vi "6762_Auto.vi"() -> ()   [LabVIEW 2017]
doc: "This VI is called when autonomous begins, and will automatically be terminated when autonomous ends. You can carry out timed or sensor driven robot movement independently without needing to return to the caller."
uses:
  <vilib>/Rock Robotics/Network Tables/NT Write Numeric Array.vi
  Robot Global Data.vi
  <vilib>/Rock Robotics/Network Tables/NT Read String.vi
panel:
  out "Current Movement, for debugging":T1 {"Y Joystick Value" scale=1.0..-1.0; "X Joystick Value" scale=-1.0..1.0}
  in  "Array of robot movements":T2(array[cluster])=[{"X Joystick Value"=0.39393939393939403, "Y Joystick Value"=0.0, "Delay (sec)"=1.0, "Movement Name"="turn"}, {"X Joystick Value"=-0.3737373737373737, "Y Joystick Value"=0.0, "Delay (sec)"=1.0, "Movement Name"="turn back"}] {"Y Joystick Value" scale=1.0..-1.0; "X Joystick Value" scale=-1.0..1.0}
  # "Be sure to right-click and choose Data Operations>>Make Current Value default if you want to save the array values with the VI"
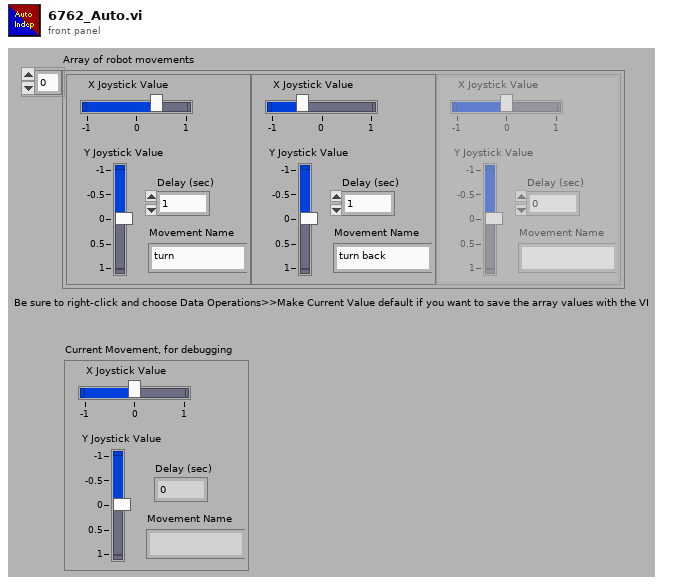
[diagram p1: front panel]
types:
  T1 = cluster{"X Joystick Value":dbl, "Y Joystick Value":dbl, "Delay (sec)":dbl, "Movement Name":string}
  T2 = cluster{"X Joystick Value":dbl, "Y Joystick Value":dbl, "Delay (sec)":dbl, "Movement Name":string}[]
  T3 = typedef "WPI_JoystickDevRef.ctl" = cluster{"Device":T4}
  T4 = typedef "WPI_JoystickDeviceEnum.ctl" = enum16{"USB 0", "USB 1", "USB 2", "USB 3", "USB 4", "USB 5"}
  T5 = enum16{"Forward", "VisionTrack00", "VisionTrackingAtEdge", "ResetTime", "TimedForward", "Stop"}
  T6 = enum16{"Start", "Vision Tracking Center", "ResetTime", "Time Forward", "drop block", "Time Reset", "Back up", "Time reset", "go Left or Right", "time Reset", "go straight", "Stop"}
  T7 = typedef "WPI_RobotDriveDevRef.ctl" = cluster{"DevStatus":errorcluster, "Motors[]":T8[], "Square Inputs":bool, "Max Output":dbl}
  T8 = typedef "WPI_MotorControlDeviceRef.ctl" = cluster{"DeviceStatus":errorcluster, "Type":T9, "PWM":cluster{"PWM Channel":T10, "DeadBand":T11}, "CAN":cluster{"Device Number":u8, "SetOutput VI Ref":variant, "GetOutput VI Ref":variant, "Enable VI Ref":variant, "Disable VI Ref":variant, "Data":variant}, "Invert":bool, "DIO PWM":cluster{"PWM \"Enable\" Channel":T10, "DIOChannel":T12, "PWM Rate":dbl}}
  T9 = typedef "WPI_MotorControlType.ctl" = enum16{"PWM", "CAN", "DIO PWM"}
  T10 = typedef "FPGA_DIOPWMChannel.ctl" = enum8{"PWM 0", "PWM 1", "PWM 2", "PWM 3", "PWM 4", "PWM 5", "PWM 6", "PWM 7", "PWM 8", "PWM 9", "PWM MXP 0", "PWM MXP 1", "PWM MXP 2", "PWM MXP 3", "PWM MXP 4", "PWM MXP 5", "PWM MXP 6", "PWM MXP 7", "PWM MXP 8", "PWM MXP 9", "Invalid"}
  T11 = typedef "WPI_PWMDeadband.ctl" = cluster{"Name":string, "maxPositivePwm":i32, "minPositivePwm":i32, "centerPwm":i32, "maxNegativePwm":i32, "minNegativePwm":i32, "angularRange":u16}
  T12 = typedef "FPGA_DIOChannel.ctl" = enum8{"DIO 0", "DIO 1", "DIO 2", "DIO 3", "DIO 4", "DIO 5", "DIO 6", "DIO 7", "DIO 8", "DIO 9", "DIO MXP 0", "DIO MXP 1", "DIO MXP 2", "DIO MXP 3", "DIO MXP 4", "DIO MXP 5", "DIO MXP 6", "DIO MXP 7", "DIO MXP 8", "DIO MXP 9", "DIO MXP 10", "DIO MXP 11", "DIO MXP 12", "DIO MXP 13", "DIO MXP 14", "DIO MXP 15", "SPI Port CS1", "SPI Port CS2", "SPI Port CS3", "SPI Port MISO", "SPI Port MOSI", "Invalid"}
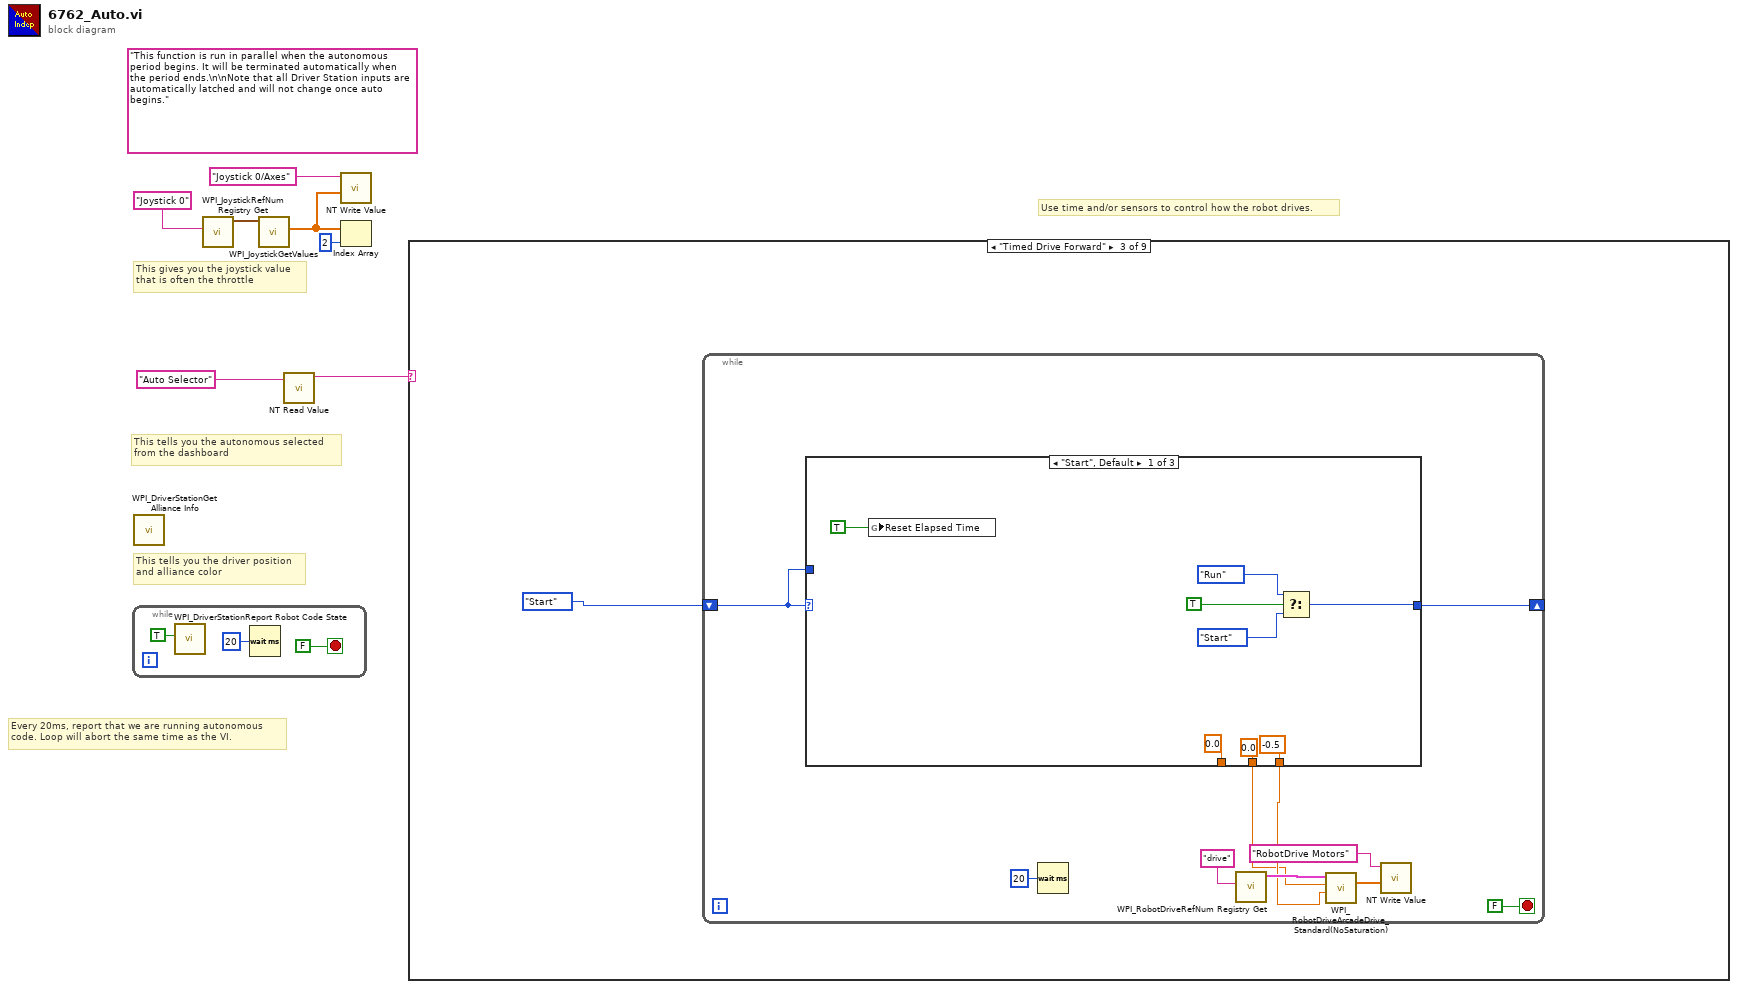
[diagram p0: block diagram]
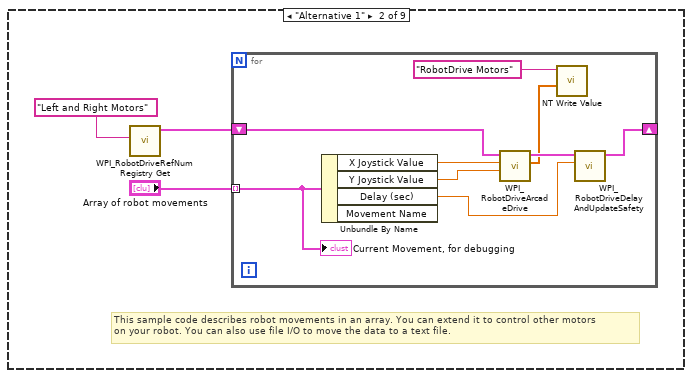
[diagram p3: hidden frame]
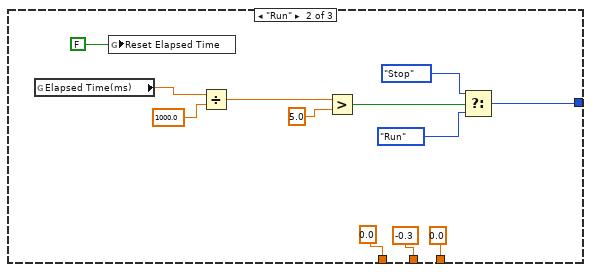
[diagram p4: hidden frame]
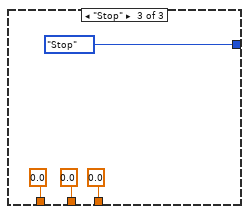
[diagram p5: hidden frame]
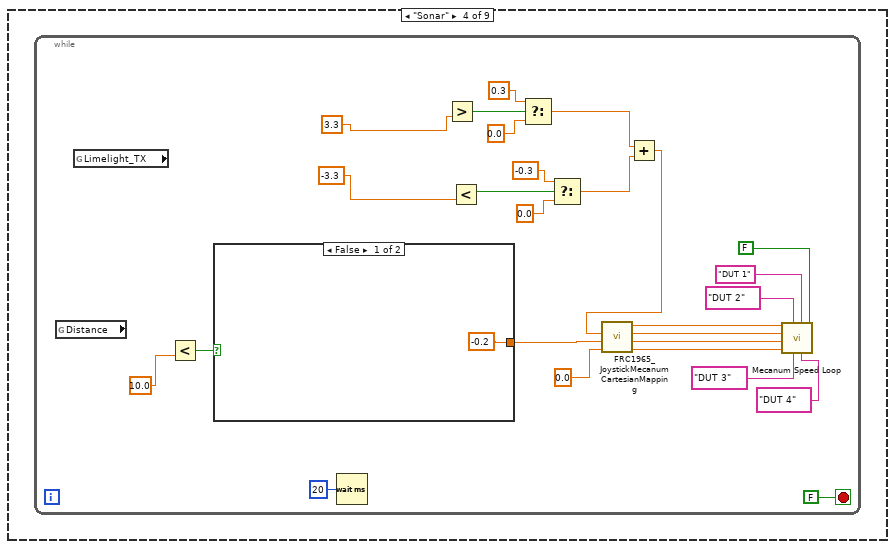
[diagram p6: hidden frame]
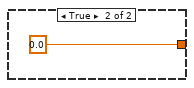
[diagram p7: hidden frame]
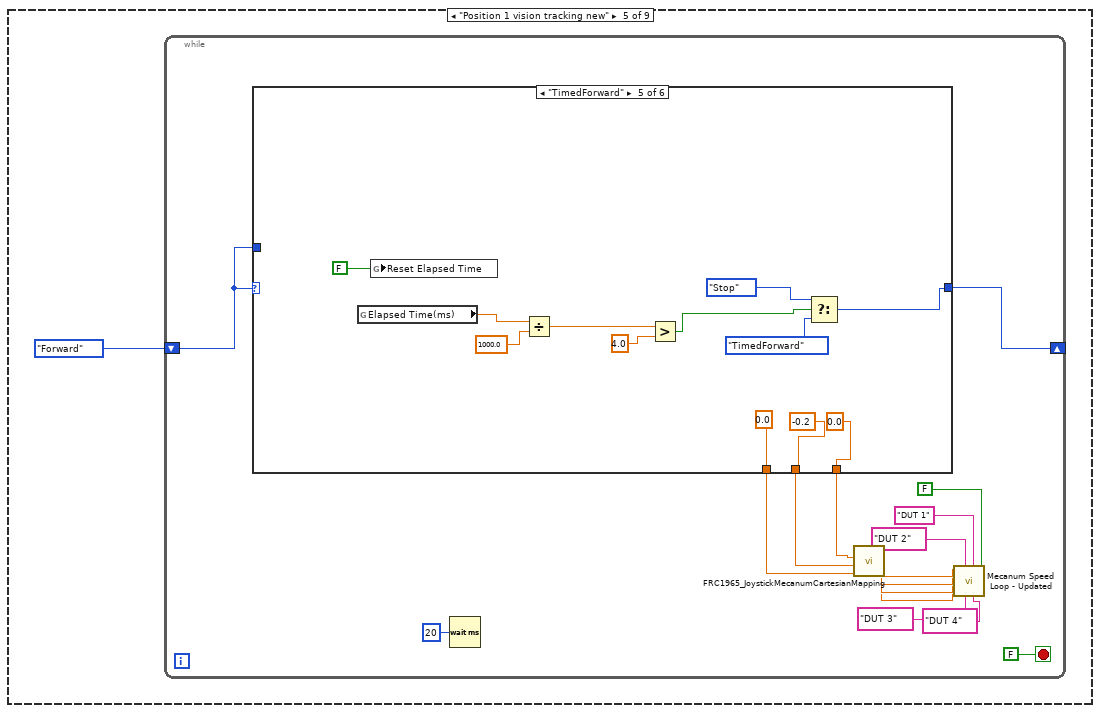
[diagram p8: hidden frame]
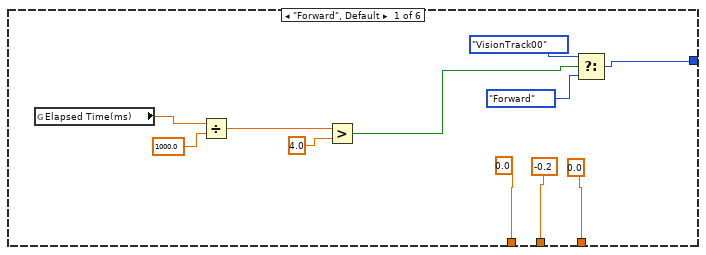
[diagram p9: hidden frame]
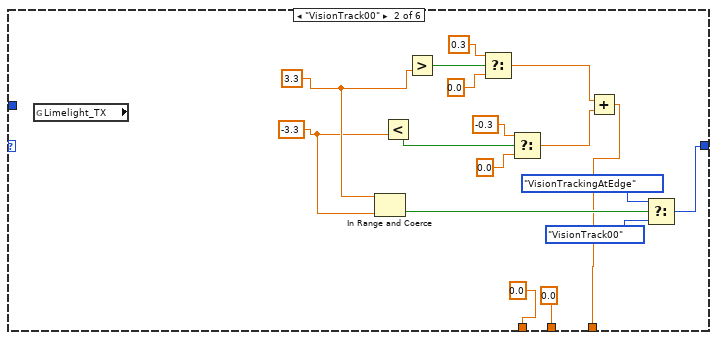
[diagram p10: hidden frame]
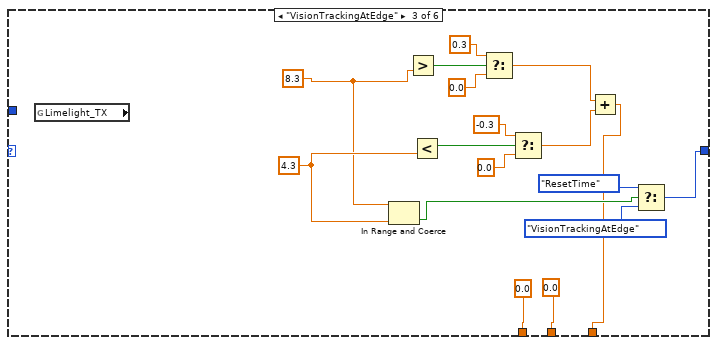
[diagram p11: hidden frame]
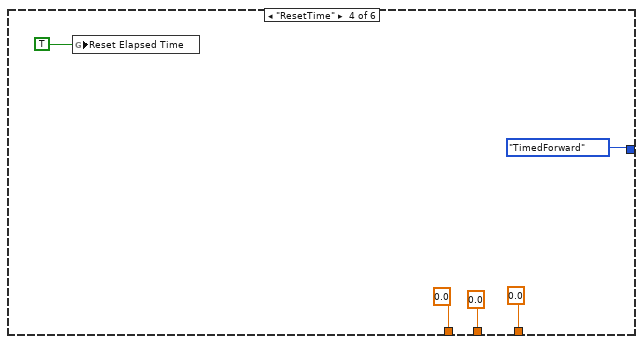
[diagram p12: hidden frame]
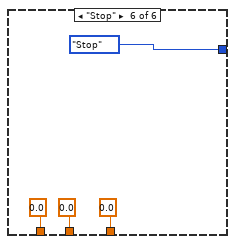
[diagram p13: hidden frame]
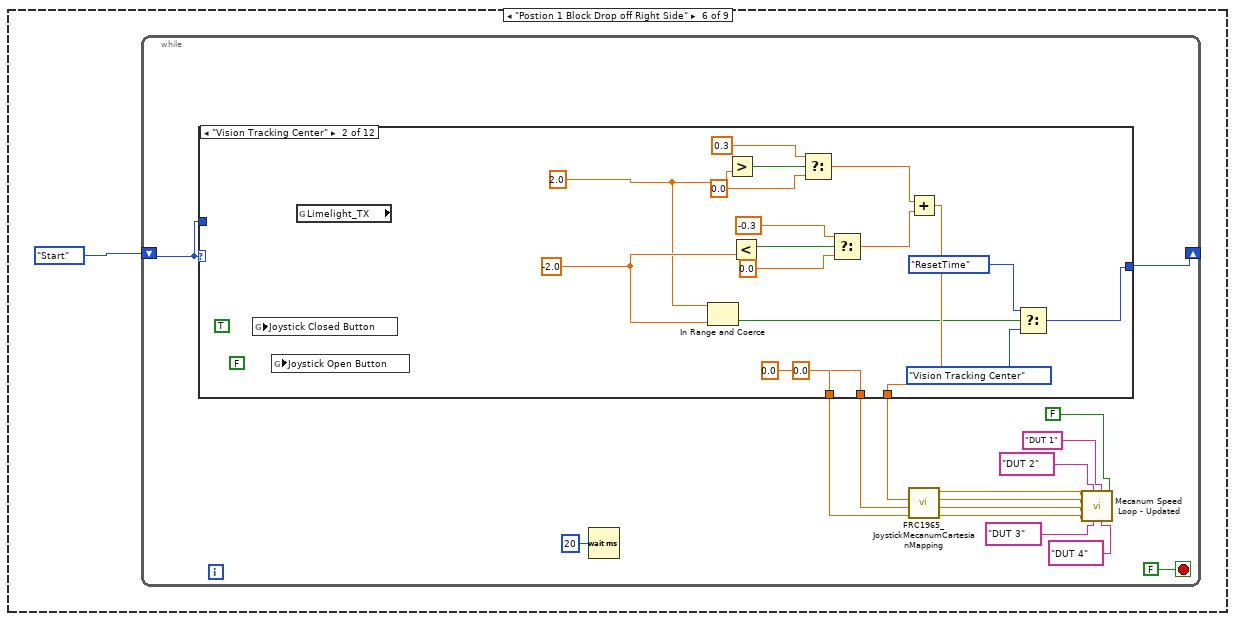
[diagram p14: hidden frame]
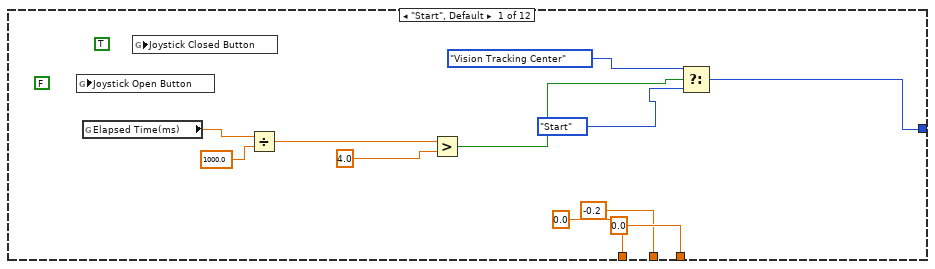
[diagram p15: hidden frame]
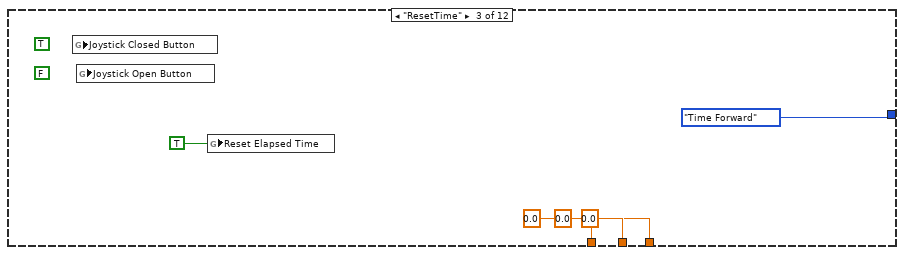
[diagram p16: hidden frame]
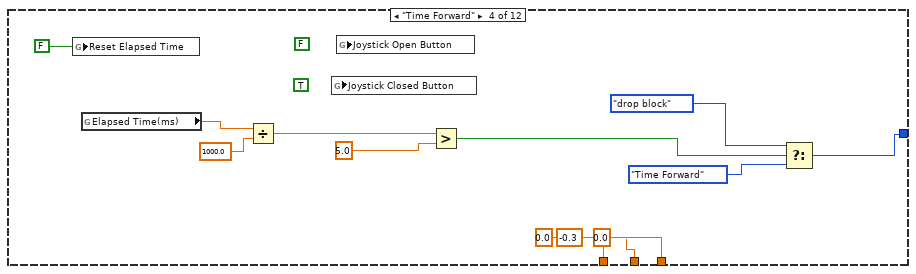
[diagram p17: hidden frame]
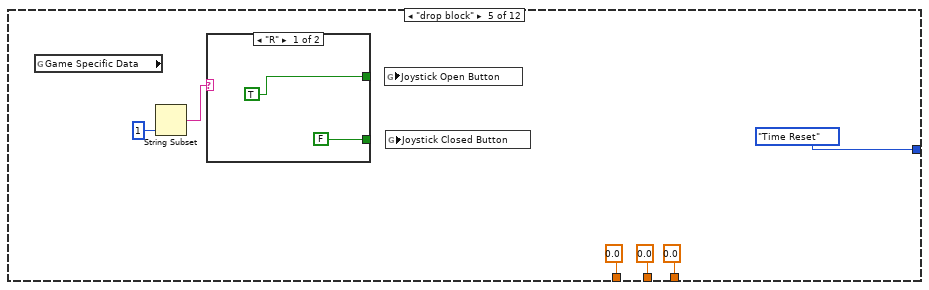
[diagram p18: hidden frame]
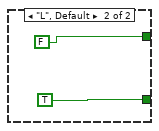
[diagram p19: hidden frame]
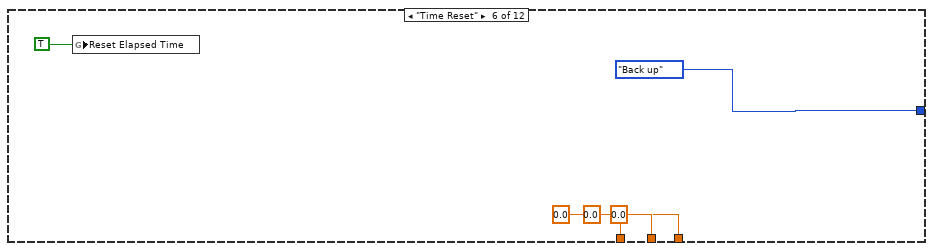
[diagram p20: hidden frame]
diagram:
  (unwired) "This function is run in parallel when the autonomous period begins. It will be terminated automatically when the period ends.\n\nNote that all Driver Station inputs are automatically latched and will not change once auto begins."
  # "Use time and/or sensors to control how the robot drives."
  # "This tells you the autonomous selected\nfrom the dashboard"
  # "Every 20ms, report that we are running autonomous\ncode. Loop will abort the same time as the VI."
  # "This gives you the joystick value\nthat is often the throttle"
  # "This tells you the driver position\nand alliance color"
  n1 = while {
    stop <- FALSE stop-if-true
    n2 = call <vilib>:"WPI_DriverStationReport Robot Code State.vi"("Autonomous"=TRUE) -> ()  [unwired: 10 in, 1 out]
    n3 = Wait (ms)(milliseconds to wait=u32 20) -> ()  [unwired: 1 out]
  }
  n4 = call <vilib>:"WPI_DriverStationGet Alliance Info.vi"() -> ()  [unwired: 12 out]
  n5 = call <vilib>:"WPI_JoystickRefNum Registry Get.vi"("refnum name"="Joystick 0") -> ("JoystickDevRef"=w6:T3)  [unwired: 1 in, 9 out]
  n6 = call <vilib>:"WPI_JoystickGetValues.vi"("JoystickDevRef"=w6) -> ("Axes"=w2:dbl[])  [unwired: 6 in, 4 out]
  n7 = call-poly <vilib>:"NT Read Value.vi"("Name"="Auto Selector") -> ("String"=w3:string)  [unwired: 9 in, 1 out]
  n8 = call-poly <vilib>:"NT Write Value.vi"("Numeric Array"=w2, "Name"="Joystick 0/Axes") -> ()  [unwired: 9 in, 1 out]
  n9 = Index Array(array=w2, index=2) -> ()  [unwired: 1 out]
  n10 = case shown="\"Timed Drive Forward\"" w3 {
    frame Default {
      # "You can put your main auto here, or you can right-click on the case and make any\nother frame be the default case."
      # "This is the frame that will execute if no selection is made, or if it is not recognized"
    }
    frame "Alternative 1" {
      # "This sample code describes robot movements in an array. You can extend it to control other motors\non your robot. You can also use file I/O to move the data to a text file."
      n11 = call <vilib>:"WPI_RobotDriveRefNum Registry Get.vi"("refnum name"="Left and Right Motors") -> ("RobotDriveDevRef"=w12:T7)  [unwired: 1 in, 9 out]
      n12 = for {
        shift-right: [w20] -> _
        shift-left: w12 -> [w21]
        tunnel: "Array of robot movements" -> [w16] mode=indexing
        n13 = Unbundle By Name(w16) -> ("X Joystick Value"=w19:dbl, "Y Joystick Value"=w18:dbl, "Delay (sec)"=w17:dbl)  [unwired: 1 out]
        n14 = call-poly <vilib>:"WPI_RobotDriveArcadeDrive.vi"("Y axis value"=w18, "X axis value"=w19, "RobotDriveDevRef"=w21) -> ("Motor Values"=w14:dbl[], "RobotDriveDevRef"=w22:T7)  [unwired: 1 in, 6 out]
        n15 = call-poly <vilib>:"NT Write Value.vi"("Numeric Array"=w14, "Name"="RobotDrive Motors") -> ()  [unwired: 9 in, 1 out]
        n16 = call <vilib>:"WPI_RobotDriveDelayAndUpdateSafety.vi"("Delay (s)"=w17, "RobotDriveDevRef"=w22) -> ("RobotDriveDevRef 2"=w20:T7)  [unwired: 8 in, 1 out]
        "Current Movement, for debugging" <- w16
      }
    }
    frame "Timed Drive Forward" {
      n17 = while {
        shift-right: [w33] -> _
        shift-left: enum16{"Start", "Run", "Stop"}."Start" ("Enum") -> [w32]
        stop <- FALSE stop-if-true
        n18 = case shown="\"Start\", Default" w32 {
          tunnel: [0.0 ("X") 0.0 ("X") 0.0 ("X")] -> _
          tunnel: [0.0 ("X") -0.3 ("X") 0.0 ("X")] -> w24
          tunnel: [-0.5 ("X") 0.0 ("X") 0.0 ("X")] -> w25
          tunnel: [w35 w48 enum16{"Start", "Run", "Stop"}."Stop" ("Enum")] -> w33
          tunnel: w32 -> [_ _ _]
          frame "Start", Default {
            n19 = global write "Robot Global Data.vi" "Reset Elapsed Time"(TRUE ("Reset Elapsed Time")) -> ()
            n20 = Select(t=enum16{"Start", "Run", "Stop"}."Run" ("Enum"), s=TRUE, f=enum16{"Start", "Run", "Stop"}."Start" ("Enum")) -> (s? t:f=w35:enum16{"Start", "Run", "Stop"})
          }
          frame "Run" {
            n21 = global read "Robot Global Data.vi" "Elapsed Time(ms)"() -> (w46:dbl)
            n22 = global write "Robot Global Data.vi" "Reset Elapsed Time"(FALSE ("Reset Elapsed Time")) -> ()
            n23 = Divide(x=w46, y=1000.0) -> (x/y=w47:dbl)
            n24 = Greater?(x=w47, y=5.0) -> (0:w43:bool)
            n25 = Select(t=enum16{"Start", "Run", "Stop"}."Stop" ("Enum"), s=w43, f=enum16{"Start", "Run", "Stop"}."Run" ("Enum")) -> (s? t:f=w48:enum16{"Start", "Run", "Stop"})
          }
          frame "Stop" {
          }
        }
        n26 = Wait (ms)(milliseconds to wait=u32 20) -> ()  [unwired: 1 out]
        n27 = call <vilib>:"WPI_RobotDriveRefNum Registry Get.vi"("refnum name"="drive") -> ("RobotDriveDevRef"=w28:T7)  [unwired: 1 in, 9 out]
        n28 = call <vilib>:"WPI_RobotDriveArcadeDrive_Standard(NoSaturation).vi"("Y axis value"=w25, "X axis value"=w24, "RobotDriveDevRef"=w28) -> ("Motor Values"=w27:dbl[])  [unwired: 1 in, 7 out]
        n29 = call-poly <vilib>:"NT Write Value.vi"("Numeric Array"=w27, "Name"="RobotDrive Motors") -> ()  [unwired: 9 in, 1 out]
      }
    }
    frame "Sonar" {
      n30 = while {
        stop <- FALSE stop-if-true
        n31 = global read "Robot Global Data.vi" "Distance"() -> ()  [unwired: 1 out]
        n32 = global read "Robot Global Data.vi" "Limelight_TX"() -> ()  [unwired: 1 out]
        n33 = Less?(y=10.0) -> (x < y?=w82:bool)  [unwired: 1 in]
        n34 = case shown="False" w82 {
          tunnel: [-0.2 ("y") 0.0 ("y")] -> w72
          frame False {
          }
          frame True {
          }
        }
        n35 = Wait (ms)(milliseconds to wait=u32 20) -> ()  [unwired: 1 out]
        n36 = Greater?(y=3.3 ("upper limit")) -> (0:w67:bool)  [unwired: 1 in]
        n37 = Less?(y=-3.3 ("lower limit")) -> (x < y?=w62:bool)  [unwired: 1 in]
        n38 = Select(t=0.3, s=w67, f=0.0) -> (s? t:f=w61:dbl)
        n39 = Select(t=-0.3, s=w62, f=0.0) -> (s? t:f=w60:dbl)
        n40 = Add(x=w61, y=w60) -> (x+y=w59:dbl)
        n41 = call "FRC1965_JoystickMecanumCartesianMapping.vi"("Rotation"=0.0, "Y"=w72, "X"=w59) -> ("Rear Right"=w73:dbl, "Rear Left"=w74:dbl, "Front Right"=w75:dbl, "Front Left"=w76:dbl)  [unwired: 5 in]
        n42 = call "Mecanum Speed Loop.vi"("Closed Loop Select"=FALSE, "DUT Number 4"="DUT 4" ("refnum name"), "DUT Number 1"="DUT 1" ("refnum name"), "DUT Number 3"="DUT 3" ("refnum name"), "DUT Number 2"="DUT 2" ("refnum name"), "Rear Right"=w73, "Rear Left"=w74, "Front Right"=w75, "Front Left"=w76) -> ()  [unwired: 3 in]
      }
    }
    frame "Position 1 vision tracking new" {
      n43 = while {
        shift-right: [w90] -> _
        shift-left: T5."Forward" ("State") -> [w89]
        stop <- FALSE stop-if-true
        n44 = case shown="\"TimedForward\"" w89 {
          tunnel: [-0.2 ("Y") 0.0 ("Rotation") 0.0 ("Rotation") 0.0 ("Rotation") -0.2 ("Rotation") 0.0 ("Rotation")] -> w93
          tunnel: [0.0 ("Rotation") 0.0 ("Rotation") 0.0 ("Rotation") 0.0 ("Rotation") 0.0 ("Rotation") 0.0 ("Rotation")] -> w92
          tunnel: [0.0 ("X") w117 w134 0.0 ("Rotation") 0.0 ("Rotation") 0.0 ("Rotation")] -> w91
          tunnel: [w103 w114 w131 T5."TimedForward" ("State") w153 T5."Stop" ("State")] -> w90
          tunnel: w89 -> [_ _ _ _ _ _]
          frame "Forward", Default {
            n45 = global read "Robot Global Data.vi" "Elapsed Time(ms)"() -> (w112:dbl)
            n46 = Divide(x=w112, y=1000.0) -> (x/y=w113:dbl)
            n47 = Greater?(x=w113, y=4.0) -> (0:w109:bool)
            n48 = Select(t=T5."VisionTrack00" ("State"), s=w109, f=T5."Forward" ("State")) -> (s? t:f=w103:T5)
          }
          frame "VisionTrack00" {
            w120 = -3.3 ("lower limit")
            w122 = 3.3 ("upper limit")
            n49 = global read "Robot Global Data.vi" "Limelight_TX"() -> ()  [unwired: 1 out]
            n50 = In Range and Coerce(upper limit=w122, lower limit=w120) -> (In Range?=w121:bool)  [unwired: 1 in, 1 out]
            n51 = Less?(y=w120) -> (x < y?=w125:bool)  [unwired: 1 in]
            n52 = Greater?(y=w122) -> (0:w130:bool)  [unwired: 1 in]
            n53 = Select(t=0.3, s=w130, f=0.0) -> (s? t:f=w124:dbl)
            n54 = Select(t=-0.3, s=w125, f=0.0) -> (s? t:f=w123:dbl)
            n55 = Add(x=w124, y=w123) -> (x+y=w117:dbl)
            n56 = Select(t=T5."VisionTrackingAtEdge" ("State"), s=w121, f=T5."VisionTrack00" ("State")) -> (s? t:f=w114:T5)
          }
          frame "VisionTrackingAtEdge" {
            w138 = 4.3 ("lower limit")
            w137 = 8.3 ("upper limit")
            n57 = global read "Robot Global Data.vi" "Limelight_TX"() -> ()  [unwired: 1 out]
            n58 = In Range and Coerce(upper limit=w137, lower limit=w138) -> (In Range?=w139:bool)  [unwired: 1 in, 1 out]
            n59 = Greater?(y=w137) -> (0:w147:bool)  [unwired: 1 in]
            n60 = Less?(y=w138) -> (x < y?=w142:bool)  [unwired: 1 in]
            n61 = Select(t=0.3, s=w147, f=0.0) -> (s? t:f=w141:dbl)
            n62 = Select(t=-0.3, s=w142, f=0.0) -> (s? t:f=w140:dbl)
            n63 = Add(x=w141, y=w140) -> (x+y=w134:dbl)
            n64 = Select(t=T5."ResetTime" ("State"), s=w139, f=T5."VisionTrackingAtEdge" ("State")) -> (s? t:f=w131:T5)
          }
          frame "ResetTime" {
            n65 = global write "Robot Global Data.vi" "Reset Elapsed Time"(TRUE ("Reset Elapsed Time")) -> ()
          }
          frame "TimedForward" {
            n66 = global read "Robot Global Data.vi" "Elapsed Time(ms)"() -> (w163:dbl)
            n67 = global write "Robot Global Data.vi" "Reset Elapsed Time"(FALSE ("Reset Elapsed Time")) -> ()
            n68 = Divide(x=w163, y=1000.0) -> (x/y=w164:dbl)
            n69 = Greater?(x=w164, y=4.0) -> (0:w160:bool)
            n70 = Select(t=T5."Stop" ("State"), s=w160, f=T5."TimedForward" ("State")) -> (s? t:f=w153:T5)
          }
          frame "Stop" {
          }
        }
        n71 = Wait (ms)(milliseconds to wait=u32 20) -> ()  [unwired: 1 out]
        n72 = call "FRC1965_JoystickMecanumCartesianMapping.vi"("Rotation"=w92, "Y"=w93, "X"=w91) -> ("Rear Right"=w99:dbl, "Rear Left"=w100:dbl, "Front Right"=w101:dbl, "Front Left"=w102:dbl)  [unwired: 5 in]
        n73 = call "Mecanum Speed Loop - Updated.vi"("Closed Loop Select"=FALSE, "DUT Number 4"="DUT 4" ("refnum name"), "DUT Number 1"="DUT 1" ("refnum name"), "DUT Number 3"="DUT 3" ("refnum name"), "DUT Number 2"="DUT 2" ("refnum name"), "Rear Right"=w99, "Rear Left"=w100, "Front Right"=w101, "Front Left"=w102) -> ()  [unwired: 3 in]
      }
    }
    frame "Postion 1 Block Drop off Right Side" {
      n74 = while {
        shift-right: [w185] -> _
        shift-left: T6."Start" ("Drop Off Block") -> [w181]
        stop <- FALSE stop-if-true
        n75 = case shown="\"Vision Tracking Center\"" w181 {
          tunnel: [w190 w199 T6."Time Forward" ("Drop Off Block") w223 T6."Time Reset" ("Drop Off Block") T6."Back up" ("Drop Off Block") w250 T6."go Left or Right" ("Drop Off Block") w266 T6."go straight" ("Drop Off Block") w284 T6."Stop" ("Drop Off Block")] -> w185
          tunnel: [0.0 ("X") w201 0.0 ("X") 0.0 ("X") 0.0 ("X") 0.0 ("X") 0.0 ("X") 0.0 ("X") 0.3 ("X") 0.0 ("X") 0.0 ("X") 0.0 ("X")] -> w184
          tunnel: [-0.2 ("X") 0.0 ("X") 0.0 ("X") -0.3 ("X") 0.0 ("X") 0.0 ("X") 0.2 ("X") 0.0 ("X") 0.0 ("X") 0.0 ("X") -0.8 ("X") 0.0 ("X")] -> w183
          tunnel: [0.0 ("X") 0.0 ("X") 0.0 ("X") 0.0 ("X") 0.0 ("X") 0.0 ("X") 0.0 ("X") 0.0 ("X") 0.0 ("X") 0.0 ("X") 0.0 ("X") 0.0 ("X")] -> w182
          tunnel: w181 -> [_ _ _ _ _ _ _ _ _ _ _ _]
          frame "Start", Default {
            (unwired) FALSE ("Joystick Closed Button")
            (unwired) TRUE ("Joystick Closed Button")
            n76 = global read "Robot Global Data.vi" "Joystick Open Button"() -> ()  [unwired: 1 in]
            n77 = global read "Robot Global Data.vi" "Elapsed Time(ms)"() -> (w195:dbl)
            n78 = global read "Robot Global Data.vi" "Joystick Closed Button"() -> ()  [unwired: 1 in]
            n79 = Divide(x=w195, y=1000.0) -> (x/y=w196:dbl)
            n80 = Greater?(x=w196, y=4.0) -> (0:w192:bool)
            n81 = Select(t=T6."Vision Tracking Center" ("Drop Off Block"), s=w192, f=T6."Start" ("Drop Off Block")) -> (s? t:f=w190:T6)
          }
          frame "Vision Tracking Center" {
            (unwired) FALSE ("Joystick Closed Button")
            (unwired) TRUE ("Joystick Closed Button")
            w203 = -2.0 ("lower limit")
            w202 = 2.0 ("upper limit")
            n82 = global read "Robot Global Data.vi" "Joystick Closed Button"() -> ()  [unwired: 1 in]
            n83 = global read "Robot Global Data.vi" "Joystick Open Button"() -> ()  [unwired: 1 in]
            n84 = global read "Robot Global Data.vi" "Limelight_TX"() -> ()  [unwired: 1 out]
            n85 = In Range and Coerce(upper limit=w202, lower limit=w203) -> (In Range?=w197:bool)  [unwired: 1 in, 1 out]
            n86 = Greater?(y=w202) -> (0:w211:bool)  [unwired: 1 in]
            n87 = Less?(y=w203) -> (x < y?=w206:bool)  [unwired: 1 in]
            n88 = Select(t=0.3, s=w211, f=0.0) -> (s? t:f=w205:dbl)
            n89 = Select(t=-0.3, s=w206, f=0.0) -> (s? t:f=w204:dbl)
            n90 = Add(x=w205, y=w204) -> (x+y=w201:dbl)
            n91 = Select(t=T6."ResetTime" ("Drop Off Block"), s=w197, f=T6."Vision Tracking Center" ("Drop Off Block")) -> (s? t:f=w199:T6)
          }
          frame "ResetTime" {
            (unwired) FALSE ("Joystick Closed Button")
            (unwired) TRUE ("Joystick Closed Button")
            n92 = global read "Robot Global Data.vi" "Joystick Closed Button"() -> ()  [unwired: 1 in]
            n93 = global read "Robot Global Data.vi" "Joystick Open Button"() -> ()  [unwired: 1 in]
            n94 = global write "Robot Global Data.vi" "Reset Elapsed Time"(TRUE ("Reset Elapsed Time")) -> ()
          }
          frame "Time Forward" {
            (unwired) FALSE ("Joystick Closed Button")
            (unwired) TRUE ("Joystick Closed Button")
            n95 = global write "Robot Global Data.vi" "Reset Elapsed Time"(FALSE ("Reset Elapsed Time")) -> ()
            n96 = global read "Robot Global Data.vi" "Elapsed Time(ms)"() -> (w228:dbl)
            n97 = Divide(x=w228, y=1000.0) -> (x/y=w229:dbl)
            n98 = global read "Robot Global Data.vi" "Joystick Closed Button"() -> ()  [unwired: 1 in]
            n99 = global read "Robot Global Data.vi" "Joystick Open Button"() -> ()  [unwired: 1 in]
            n100 = Greater?(x=w229, y=5.0) -> (0:w222:bool)
            n101 = Select(t=T6."drop block" ("Drop Off Block"), s=w222, f=T6."Time Forward" ("Drop Off Block")) -> (s? t:f=w223:T6)
          }
          frame "drop block" {
            n102 = global read "Robot Global Data.vi" "Game Specific Data"() -> ()  [unwired: 1 out]
            n103 = String Subset(length (rest)=1 ("length (rest)")) -> (substring=w232:string)  [unwired: 2 in]
            n104 = case shown="\"R\"" w232 {
              tunnel: [TRUE FALSE] -> _
              tunnel: [FALSE ("Joystick Closed Button") TRUE ("Joystick Closed Button")] -> _
              frame "R" {
              }
              frame "L", Default {
              }
            }
            n105 = global read "Robot Global Data.vi" "Joystick Open Button"() -> ()  [unwired: 1 in]
            n106 = global read "Robot Global Data.vi" "Joystick Closed Button"() -> ()  [unwired: 1 in]
          }
          frame "Time Reset" {
            n107 = global write "Robot Global Data.vi" "Reset Elapsed Time"(TRUE ("Reset Elapsed Time")) -> ()
          }
          frame "Back up" {
            n108 = global read "Robot Global Data.vi" "Elapsed Time(ms)"() -> (w255:dbl)
            n109 = global write "Robot Global Data.vi" "Reset Elapsed Time"(FALSE ("Reset Elapsed Time")) -> ()
            n110 = Divide(x=w255, y=1000.0) -> (x/y=w256:dbl)
            n111 = Greater?(x=w256, y=2.0) -> (0:w249:bool)
            n112 = Select(t=T6."Time reset" ("Drop Off Block"), s=w249, f=T6."Back up" ("Drop Off Block")) -> (s? t:f=w250:T6)
          }
          frame "Time reset" {
            n113 = global write "Robot Global Data.vi" "Reset Elapsed Time"(TRUE ("Reset Elapsed Time")) -> ()
          }
          frame "go Left or Right" {
            n114 = global write "Robot Global Data.vi" "Reset Elapsed Time"(FALSE ("Reset Elapsed Time")) -> ()
            n115 = global read "Robot Global Data.vi" "Elapsed Time(ms)"() -> (w272:dbl)
            n116 = Divide(x=w272, y=1000.0) -> (x/y=w273:dbl)
            n117 = Greater?(x=w273, y=3.0) -> (0:w267:bool)
            n118 = Select(t=T6."time Reset" ("Drop Off Block"), s=w267, f=T6."go Left or Right" ("Drop Off Block")) -> (s? t:f=w266:T6)
          }
          frame "time Reset" {
            n119 = global write "Robot Global Data.vi" "Reset Elapsed Time"(TRUE ("Reset Elapsed Time")) -> ()
          }
          frame "go straight" {
            n120 = global write "Robot Global Data.vi" "Reset Elapsed Time"(FALSE ("Reset Elapsed Time")) -> ()
            n121 = global read "Robot Global Data.vi" "Elapsed Time(ms)"() -> (w289:dbl)
            n122 = Divide(x=w289, y=1000.0) -> (x/y=w290:dbl)
            n123 = Greater?(x=w290, y=3.0) -> (0:w283:bool)
            n124 = Select(t=T6."Stop" ("Drop Off Block"), s=w283, f=T6."go straight" ("Drop Off Block")) -> (s? t:f=w284:T6)
          }
          frame "Stop" {
          }
        }
        n125 = Wait (ms)(milliseconds to wait=u32 20) -> ()  [unwired: 1 out]
        n126 = call "FRC1965_JoystickMecanumCartesianMapping.vi"("Rotation"=w182, "Y"=w183, "X"=w184) -> ("Rear Right"=w174:dbl, "Rear Left"=w173:dbl, "Front Right"=w172:dbl, "Front Left"=w171:dbl)  [unwired: 5 in]
        n127 = call "Mecanum Speed Loop - Updated.vi"("Closed Loop Select"=FALSE, "DUT Number 4"="DUT 4" ("refnum name"), "DUT Number 1"="DUT 1" ("refnum name"), "DUT Number 3"="DUT 3" ("refnum name"), "DUT Number 2"="DUT 2" ("refnum name"), "Rear Right"=w174, "Rear Left"=w173, "Front Right"=w172, "Front Left"=w171) -> ()  [unwired: 3 in]
      }
    }
    frame "Postion 1 Left side Drop off" {
      n128 = while {
        shift-right: [w312] -> _
        shift-left: T6."Start" ("Drop Off Block") -> [w308]
        stop <- FALSE stop-if-true
        n129 = case shown="\"go straight\"" w308 {
          tunnel: [w317 w326 T6."Time Forward" ("Drop Off Block") w350 T6."Time Reset" ("Drop Off Block") T6."Back up" ("Drop Off Block") w377 T6."go Left or Right" ("Drop Off Block") w393 T6."go straight" ("Drop Off Block") w411 T6."Stop" ("Drop Off Block")] -> w312
          tunnel: [0.0 ("X") w328 0.0 ("X") 0.0 ("X") 0.0 ("X") 0.0 ("X") 0.0 ("X") 0.0 ("X") -0.3 ("X") 0.0 ("X") 0.0 ("X") 0.0 ("X")] -> w311
          tunnel: [-0.2 ("X") 0.0 ("X") 0.0 ("X") -0.3 ("X") 0.0 ("X") 0.0 ("X") 0.2 ("X") 0.0 ("X") 0.0 ("X") 0.0 ("X") -0.8 ("X") 0.0 ("X")] -> w310
          tunnel: [0.0 ("X") 0.0 ("X") 0.0 ("X") 0.0 ("X") 0.0 ("X") 0.0 ("X") 0.0 ("X") 0.0 ("X") 0.0 ("X") 0.0 ("X") 0.0 ("X") 0.0 ("X")] -> w309
          tunnel: w308 -> [_ _ _ _ _ _ _ _ _ _ _ _]
          frame "Start", Default {
            (unwired) TRUE ("Joystick Closed Button")
            (unwired) FALSE ("Joystick Closed Button")
            n130 = global read "Robot Global Data.vi" "Elapsed Time(ms)"() -> (w322:dbl)
            n131 = global read "Robot Global Data.vi" "Joystick Closed Button"() -> ()  [unwired: 1 in]
            n132 = global read "Robot Global Data.vi" "Joystick Open Button"() -> ()  [unwired: 1 in]
            n133 = Divide(x=w322, y=1000.0) -> (x/y=w323:dbl)
            n134 = Greater?(x=w323, y=4.0) -> (0:w319:bool)
            n135 = Select(t=T6."Vision Tracking Center" ("Drop Off Block"), s=w319, f=T6."Start" ("Drop Off Block")) -> (s? t:f=w317:T6)
          }
          frame "Vision Tracking Center" {
            (unwired) TRUE ("Joystick Closed Button")
            (unwired) FALSE ("Joystick Closed Button")
            w330 = -2.0 ("lower limit")
            w329 = 2.0 ("upper limit")
            n136 = global read "Robot Global Data.vi" "Limelight_TX"() -> ()  [unwired: 1 out]
            n137 = global read "Robot Global Data.vi" "Joystick Closed Button"() -> ()  [unwired: 1 in]
            n138 = global read "Robot Global Data.vi" "Joystick Open Button"() -> ()  [unwired: 1 in]
            n139 = In Range and Coerce(upper limit=w329, lower limit=w330) -> (In Range?=w324:bool)  [unwired: 1 in, 1 out]
            n140 = Greater?(y=w329) -> (0:w338:bool)  [unwired: 1 in]
            n141 = Less?(y=w330) -> (x < y?=w333:bool)  [unwired: 1 in]
            n142 = Select(t=0.3, s=w338, f=0.0) -> (s? t:f=w332:dbl)
            n143 = Select(t=-0.3, s=w333, f=0.0) -> (s? t:f=w331:dbl)
            n144 = Add(x=w332, y=w331) -> (x+y=w328:dbl)
            n145 = Select(t=T6."ResetTime" ("Drop Off Block"), s=w324, f=T6."Vision Tracking Center" ("Drop Off Block")) -> (s? t:f=w326:T6)
          }
          frame "ResetTime" {
            (unwired) TRUE ("Joystick Closed Button")
            (unwired) FALSE ("Joystick Closed Button")
            n146 = global read "Robot Global Data.vi" "Joystick Closed Button"() -> ()  [unwired: 1 in]
            n147 = global read "Robot Global Data.vi" "Joystick Open Button"() -> ()  [unwired: 1 in]
            n148 = global write "Robot Global Data.vi" "Reset Elapsed Time"(TRUE ("Reset Elapsed Time")) -> ()
          }
          frame "Time Forward" {
            (unwired) TRUE ("Joystick Closed Button")
            (unwired) FALSE ("Joystick Closed Button")
            n149 = global write "Robot Global Data.vi" "Reset Elapsed Time"(FALSE ("Reset Elapsed Time")) -> ()
            n150 = global read "Robot Global Data.vi" "Elapsed Time(ms)"() -> (w355:dbl)
            n151 = Divide(x=w355, y=1000.0) -> (x/y=w356:dbl)
            n152 = global read "Robot Global Data.vi" "Joystick Closed Button"() -> ()  [unwired: 1 in]
            n153 = global read "Robot Global Data.vi" "Joystick Open Button"() -> ()  [unwired: 1 in]
            n154 = Greater?(x=w356, y=5.0) -> (0:w349:bool)
            n155 = Select(t=T6."drop block" ("Drop Off Block"), s=w349, f=T6."Time Forward" ("Drop Off Block")) -> (s? t:f=w350:T6)
          }
          frame "drop block" {
            n156 = global read "Robot Global Data.vi" "Game Specific Data"() -> ()  [unwired: 1 out]
            n157 = String Subset(length (rest)=1 ("length (rest)")) -> (substring=w359:string)  [unwired: 2 in]
            n158 = case shown="\"R\", Default" w359 {
              tunnel: [FALSE TRUE] -> _
              tunnel: [TRUE FALSE] -> _
              frame "R", Default {
              }
              frame "L" {
              }
            }
            n159 = global read "Robot Global Data.vi" "Joystick Open Button"() -> ()  [unwired: 1 in]
            n160 = global read "Robot Global Data.vi" "Joystick Closed Button"() -> ()  [unwired: 1 in]
          }
          frame "Time Reset" {
            n161 = global write "Robot Global Data.vi" "Reset Elapsed Time"(TRUE ("Reset Elapsed Time")) -> ()
          }
          frame "Back up" {
            n162 = global read "Robot Global Data.vi" "Elapsed Time(ms)"() -> (w382:dbl)
            n163 = global write "Robot Global Data.vi" "Reset Elapsed Time"(FALSE ("Reset Elapsed Time")) -> ()
            n164 = Divide(x=w382, y=1000.0) -> (x/y=w383:dbl)
            n165 = Greater?(x=w383, y=2.0) -> (0:w376:bool)
            n166 = Select(t=T6."Time reset" ("Drop Off Block"), s=w376, f=T6."Back up" ("Drop Off Block")) -> (s? t:f=w377:T6)
          }
          frame "Time reset" {
            n167 = global write "Robot Global Data.vi" "Reset Elapsed Time"(TRUE ("Reset Elapsed Time")) -> ()
          }
          frame "go Left or Right" {
            n168 = global write "Robot Global Data.vi" "Reset Elapsed Time"(FALSE ("Reset Elapsed Time")) -> ()
            n169 = global read "Robot Global Data.vi" "Elapsed Time(ms)"() -> (w399:dbl)
            n170 = Divide(x=w399, y=1000.0) -> (x/y=w400:dbl)
            n171 = Greater?(x=w400, y=3.0) -> (0:w394:bool)
            n172 = Select(t=T6."time Reset" ("Drop Off Block"), s=w394, f=T6."go Left or Right" ("Drop Off Block")) -> (s? t:f=w393:T6)
          }
          frame "time Reset" {
            n173 = global write "Robot Global Data.vi" "Reset Elapsed Time"(TRUE ("Reset Elapsed Time")) -> ()
          }
          frame "go straight" {
            n174 = global write "Robot Global Data.vi" "Reset Elapsed Time"(FALSE ("Reset Elapsed Time")) -> ()
            n175 = global read "Robot Global Data.vi" "Elapsed Time(ms)"() -> (w416:dbl)
            n176 = Divide(x=w416, y=1000.0) -> (x/y=w417:dbl)
            n177 = Greater?(x=w417, y=3.0) -> (0:w410:bool)
            n178 = Select(t=T6."Stop" ("Drop Off Block"), s=w410, f=T6."go straight" ("Drop Off Block")) -> (s? t:f=w411:T6)
          }
          frame "Stop" {
          }
        }
        n179 = Wait (ms)(milliseconds to wait=u32 20) -> ()  [unwired: 1 out]
        n180 = call "FRC1965_JoystickMecanumCartesianMapping.vi"("Rotation"=w309, "Y"=w310, "X"=w311) -> ("Rear Right"=w301:dbl, "Rear Left"=w300:dbl, "Front Right"=w299:dbl, "Front Left"=w298:dbl)  [unwired: 5 in]
        n181 = call "Mecanum Speed Loop - Updated.vi"("Closed Loop Select"=FALSE, "DUT Number 4"="DUT 4" ("refnum name"), "DUT Number 1"="DUT 1" ("refnum name"), "DUT Number 3"="DUT 3" ("refnum name"), "DUT Number 2"="DUT 2" ("refnum name"), "Rear Right"=w301, "Rear Left"=w300, "Front Right"=w299, "Front Left"=w298) -> ()  [unwired: 3 in]
      }
    }
    frame "Alternative 2" {
      w424 = "RobotDrive Motors" ("Name")
      # "This is some simple sample code to drive your robot curving one direction and then the other."
      # "stand still"
      # "other way for 0.5 second"
      # "turn for 1 second"
      n182 = call <vilib>:"WPI_RobotDriveRefNum Registry Get.vi"("refnum name"="Left and Right Motors") -> ("RobotDriveDevRef"=w440:T7)  [unwired: 1 in, 9 out]
      n183 = call-poly <vilib>:"WPI_RobotDriveArcadeDrive.vi"("Y axis value"=0.5 ("X axis value"), "X axis value"=-0.25, "RobotDriveDevRef"=w440) -> ("Motor Values"=w423:dbl[], "RobotDriveDevRef"=w433:T7)  [unwired: 1 in, 6 out]
      n184 = call-poly <vilib>:"NT Write Value.vi"("Numeric Array"=w423, "Name"=w424) -> ()  [unwired: 9 in, 1 out]
      n185 = call <vilib>:"WPI_RobotDriveDelayAndUpdateSafety.vi"("Delay (s)"=1.0, "RobotDriveDevRef"=w433) -> ("RobotDriveDevRef 2"=w434:T7)  [unwired: 8 in, 1 out]
      n186 = call-poly <vilib>:"WPI_RobotDriveArcadeDrive.vi"("Y axis value"=-0.25 ("X axis value"), "X axis value"=0.5, "RobotDriveDevRef"=w434) -> ("Motor Values"=w425:dbl[], "RobotDriveDevRef"=w435:T7)  [unwired: 1 in, 6 out]
      n187 = call-poly <vilib>:"NT Write Value.vi"("Numeric Array"=w425, "Name"=w424) -> ()  [unwired: 9 in, 1 out]
      n188 = call <vilib>:"WPI_RobotDriveDelayAndUpdateSafety.vi"("Delay (s)"=0.5, "RobotDriveDevRef"=w435) -> ("RobotDriveDevRef 2"=w436:T7)  [unwired: 8 in, 1 out]
      n189 = call-poly <vilib>:"WPI_RobotDriveArcadeDrive.vi"("Y axis value"=0.0 ("X axis value"), "X axis value"=0.0, "RobotDriveDevRef"=w436) -> ("Motor Values"=w426:dbl[])  [unwired: 1 in, 7 out]
      n190 = call-poly <vilib>:"NT Write Value.vi"("Numeric Array"=w426, "Name"=w424) -> ()  [unwired: 9 in, 1 out]
    }
    frame "Your Turn" {
    }
  }
